vi "Test Scrubber Found For All Date Types.vi"(8 "error in (no error)":errorcluster) -> (0 "error out":errorcluster)   [LabVIEW 2020, in "Scrubber.Tests.lvclass"]
uses:
  Scrubber.Tests.lvclass
  <vilib>/addons/_JKI Toolkits/Caraya/classes/Assert/Assert True.vi
  Scrubber.Tests.lvclass/Scrubber.Tests.ctl
  <vilib>/addons/_JKI Toolkits/Caraya/classes/Test/Test.lvclass
  <vilib>/addons/_JKI Toolkits/Caraya/classes/Assert/Assert.lvclass
  Source/Approval Tests/Date Scrubber/Date Scrubber.lvclass
  <vilib>/addons/_JKI Toolkits/Caraya/classes/Assert/Assert False.vi
panel:
  out "Scrubbers Missing":string[](array[string])
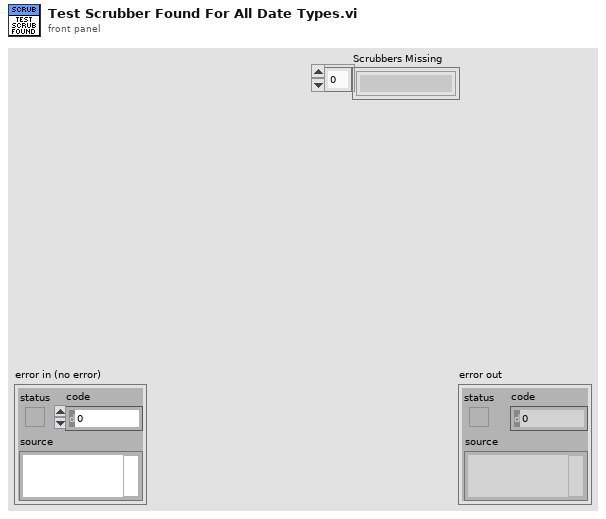
[diagram p1: front panel]
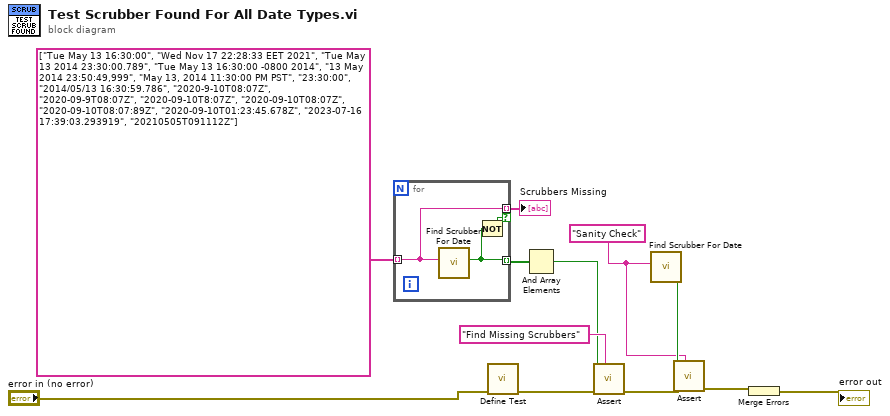
[diagram p0: block diagram]
diagram:
  w1 = "Sanity Check"
  n1 = for {
    tunnel: string[] ["Tue May 13 16:30:00", "Wed Nov 17 22:28:33 EET 2021", "Tue May 13 2014 23:30:00.789", "Tue May 13 16:30:00 -0800 2014", "13 May 2014 23:50:49,999", "May 13, 2014 11:30:00 PM PST", "23:30:00", "2014/05/13 16:30:59.786", "2020-9-10T08:07Z", "2020-09-9T08:07Z", "2020-09-10T8:07Z", "2020-09-10T08:07Z", "2020-09-10T08:07:89Z", "2020-09-10T01:23:45.678Z", "2023-07-16 17:39:03.293919", "20210505T091112Z"] ("subarray") -> [w15] mode=indexing
    tunnel: [w14] -> w7 mode=indexing
    tunnel: [w15] -> w5 mode=indexing if=w13
    n2 = call "Find Scrubber For Date.vi"("Sample Date"=w15) -> ("Found?"=w14:bool)  [unwired: 8 in, 2 out]
    n3 = Not(x=w14) -> (.not. x?=w13:bool)
  }
  "Scrubbers Missing" <- w5
  n4 = call <vilib>:"Define Test.vi"("error in (no error)"="error in (no error)") -> ("error out"=w11:errorcluster)  [unwired: 9 in, 1 out]
  n5 = And Array Elements(Boolean array=w7) -> (logical AND=w6:bool)
  n6 = call-poly <vilib>:"Assert.vi"("Label"="Find Missing Scrubbers" ("Label (VI Title)"), "error in (no error)"=w11, "True?"=w6) -> ("error out"=w4:errorcluster)  [unwired: 7 in, 1 out]
  n7 = call "Find Scrubber For Date.vi"("Sample Date"=w1) -> ("Found?"=w2:bool)  [unwired: 8 in, 2 out]
  n8 = call-poly <vilib>:"Assert.vi"("Label"=w1, "error in (no error)"=w4, "False?"=w2) -> ("error out"=w3:errorcluster)  [unwired: 7 in, 1 out]
  n9 = Merge Errors(w3) -> (→"error out":errorcluster)
